vi "Parse ITX String.vi"(8 "error in (no error)":errorcluster, 11 "ITX String":string) -> (0 "error out":errorcluster, 1 "Commands":string, 2 "Notes":string, 3 "Array":T1[](array[typedef]))   [LabVIEW 2019, in "Data.ITX.lvclass"]
uses:
  Data.ITX.lvclass
  Data/Typedefs/Dictionary--cluster.ctl
  Data/Data.lvclass
  _OpenG.lib/string/string.llb/Trim Whitespace (String)__ogtk.vi
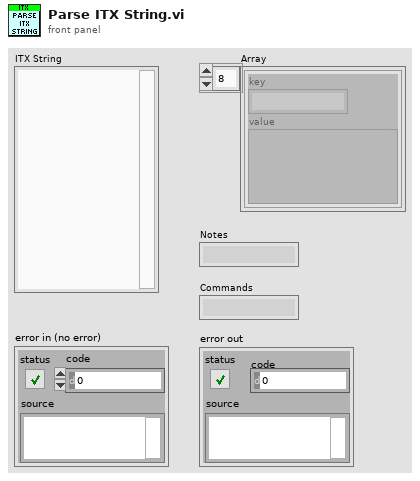
[diagram p1: front panel]
types:
  T1 = typedef "Data.lvclass/Dictionary--cluster.ctl" = cluster{"key":string, "value":variant}
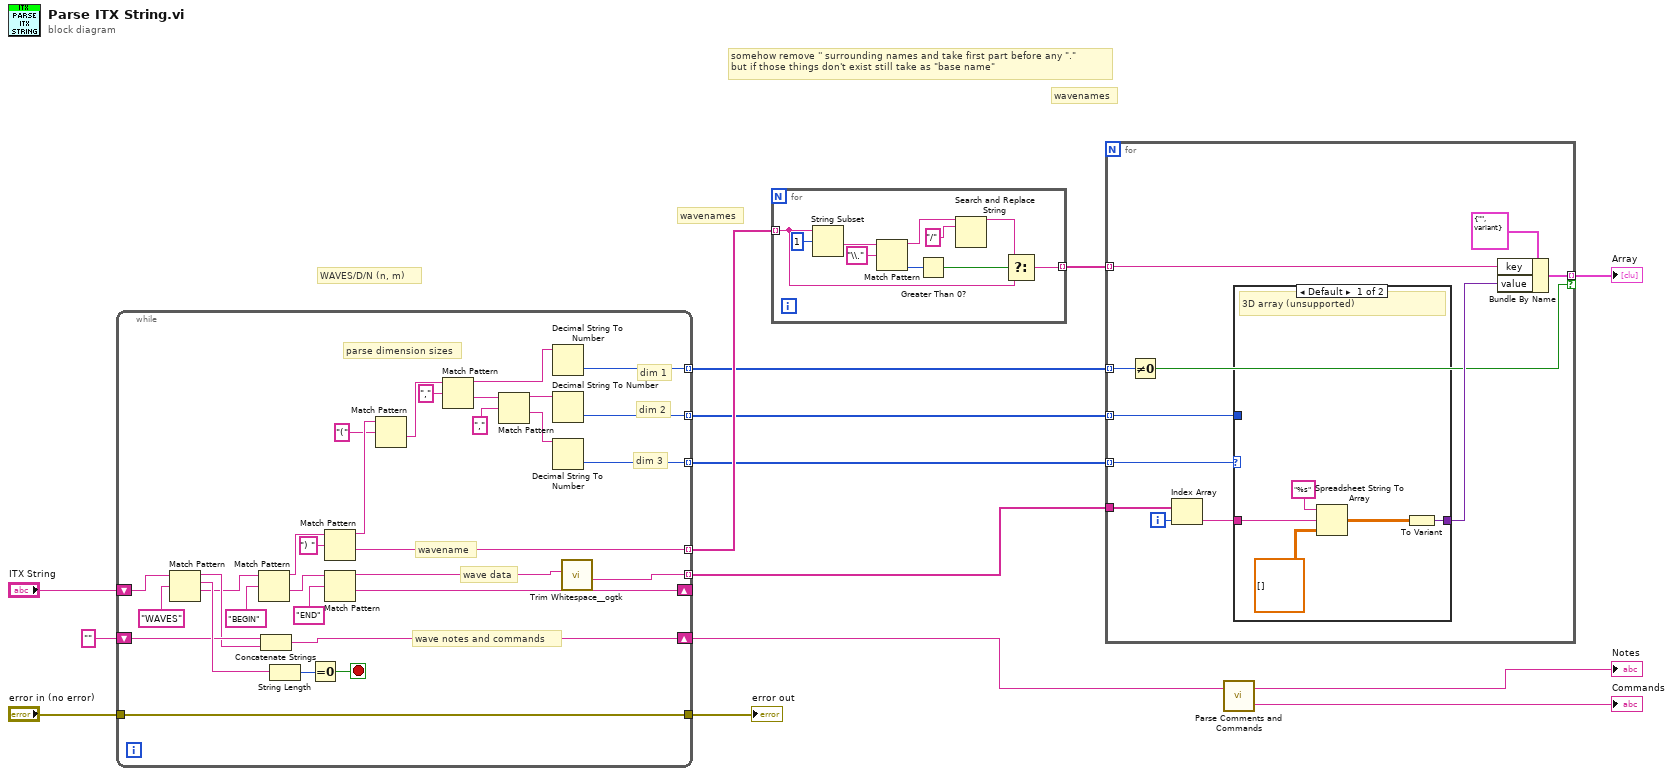
[diagram p0: block diagram]
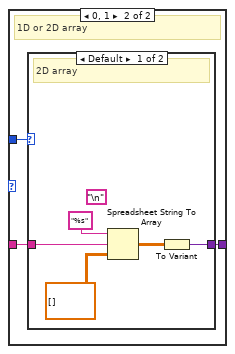
[diagram p2: hidden frame]
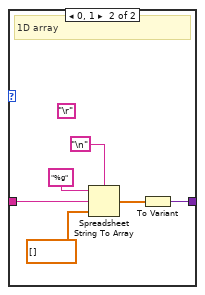
[diagram p3: hidden frame]
diagram:
  # "wavenames"
  # "wavenames"
  # "somehow remove '' surrounding names and take first part before any \".\"\nbut if those things don't exist still take as \"base name\""
  # "WAVES/D/N (n, m)"
  n1 = while {
    tunnel: [w20] -> w10 mode=indexing
    shift-right: [w44] -> _
    shift-left: "ITX String" -> [w32]
    tunnel: [w40] -> w8 mode=indexing
    shift-right: [w35] -> w1
    shift-left: "" ("regular expression") -> [w34]
    tunnel: [w30] -> w11
    tunnel: "error in (no error)" -> [w30]
    tunnel: [w22] -> w5 mode=indexing
    tunnel: [w24] -> w6 mode=indexing
    tunnel: [w15] -> w7 mode=indexing
    stop <- w41 stop-if-true
    # "dim 3"
    # "dim 2"
    # "dim 1"
    # "wave data"
    # "wave notes and commands"
    # "parse dimension sizes"
    # "wavename"
    n2 = Match Pattern(string=w32, regular expression="WAVES") -> (before substring=w33:string, match substring=w43:string, after substring=w29:string)  [unwired: 2 out]
    n3 = Match Pattern(string=w29, regular expression="BEGIN" ("regular expression 2")) -> (before substring=w31:string, after substring=w45:string)  [unwired: 3 out]
    n4 = Concatenate Strings(w34, w33) -> (w35:string)
    n5 = String Length(string=w43) -> (length=w42:i32)
    n6 = Equal To 0?(x=w42) -> (x = 0?=w41:bool)
    n7 = Match Pattern(string=w31, regular expression=") ") -> (before substring=w28:string, after substring=w40:string)  [unwired: 3 out]
    n8 = Match Pattern(string=w45, regular expression="END" ("regular expression 3")) -> (before substring=w21:string, after substring=w44:string)  [unwired: 3 out]
    n9 = Match Pattern(string=w28, regular expression="(") -> (after substring=w26:string)  [unwired: 4 out]
    n10 = Match Pattern(string=w26, regular expression=",") -> (before substring=w23:string, after substring=w19:string)  [unwired: 3 out]
    n11 = Match Pattern(string=w19, regular expression=",") -> (before substring=w17:string, after substring=w18:string)  [unwired: 3 out]
    n12 = Decimal String To Number(string=w23) -> (number=w22:i32)  [unwired: 2 in, 1 out]
    n13 = Decimal String To Number(string=w17) -> (number=w24:i32)  [unwired: 2 in, 1 out]
    n14 = Decimal String To Number(string=w18) -> (number=w15:i32)  [unwired: 2 in, 1 out]
    n15 = call-poly "Trim Whitespace__ogtk.vi"("String in"=w21) -> ("String out"=w20:string)  [unwired: 6 in]
  }
  "error out" <- w11
  n16 = for {
    tunnel: w8 -> [w47] mode=indexing
    tunnel: [w48] -> w9 mode=indexing
    n17 = String Subset(string=w47, offset (0)=1) -> (substring=w54:string)  [unwired: 1 in]
    n18 = Match Pattern(string=w54, regular expression="\\.") -> (before substring=w50:string, offset past match=w52:i32)  [unwired: 1 in, 2 out]
    n19 = Greater Than 0?(x=w52) -> (x > 0?=w49:bool)
    n20 = Search and Replace String(input string=w50, search string="/") -> (result string=w46:string)  [unwired: 6 in, 3 out]
    n21 = Select(t=w46, s=w49, f=w47) -> (s? t:f=w48:string)
  }
  n22 = for {
    tunnel: w10 -> [w66]
    tunnel: w9 -> [w59] mode=indexing
    tunnel: [w64] -> w12 mode=indexing if=w56
    tunnel: w5 -> [w57] mode=indexing
    tunnel: w6 -> [w61] mode=indexing
    tunnel: w7 -> [w62] mode=indexing
    i -> [w65]
    n23 = Not Equal To 0?(x=w57) -> (x != 0?=w56:bool)
    n24 = Index Array(array=w66, index=w65) -> (element=w60:string)
    n25 = case shown="Default" w62 {
      tunnel: w60 -> [w69 w73]
      tunnel: [w71 w74] -> w58
      tunnel: w61 -> [_ w72]
      frame Default {
        # "3D array (unsupported)"
        n26 = Spreadsheet String To Array(format string="%s", spreadsheet string=w69, array type (2D Dbl)=dbl[][][] []) -> (array=w68:dbl[][][])  [unwired: 1 out]
        n27 = To Variant(anything=w68) -> (Variant=w71:variant)
      }
      frame 0, 1 {
        # "1D or 2D array"
        n28 = case shown="Default" w72 {
          tunnel: [w79 w85] -> w74
          tunnel: w73 -> [w77 w84]
          frame Default {
            (unwired) "\n"
            # "2D array"
            n29 = Spreadsheet String To Array(format string="%s", spreadsheet string=w77, array type (2D Dbl)=dbl[][] []) -> (array=w76:dbl[][])  [unwired: 1 out]
            n30 = To Variant(anything=w76) -> (Variant=w79:variant)
          }
          frame 0, 1 {
            (unwired) "\r"
            # "1D array"
            n31 = Spreadsheet String To Array(delimiter (Tab)="\n", format string="%g", spreadsheet string=w84, array type (2D Dbl)=dbl[] []) -> (array=w83:dbl[])
            n32 = To Variant(anything=w83) -> (Variant=w85:variant)
          }
        }
      }
    }
    n33 = Bundle By Name(cluster=T1 {"key"="", "value"=variant} ("key-value"), "key"=w59, "value"=w58) -> (w64:T1)
  }
  "Array" <- w12
  n34 = call "Parse Comments and Commands.vi"("ITX Notes and Commands"=w1) -> ("Commands"=→"Commands":string, "Notes"=→"Notes":string)  [unwired: 1 in]
